vi "get time stamp.vi"(8 "error in (no error)":errorcluster, 10 "clockspeed":dbl, 11 "Image":T1) -> (0 "error out":errorcluster, 3 "timestamp":dbl)   [LabVIEW 2020, in "Point Grey Camera.lvclass"]
uses:
  Point Grey Camera.lvclass
  IMAQ Image.ctl
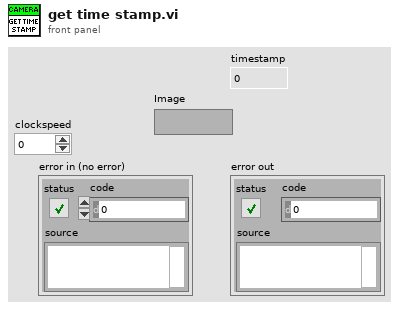
[diagram p1: front panel]
types:
  T1 = typedef "IMAQ Image.ctl" = refnum<image>
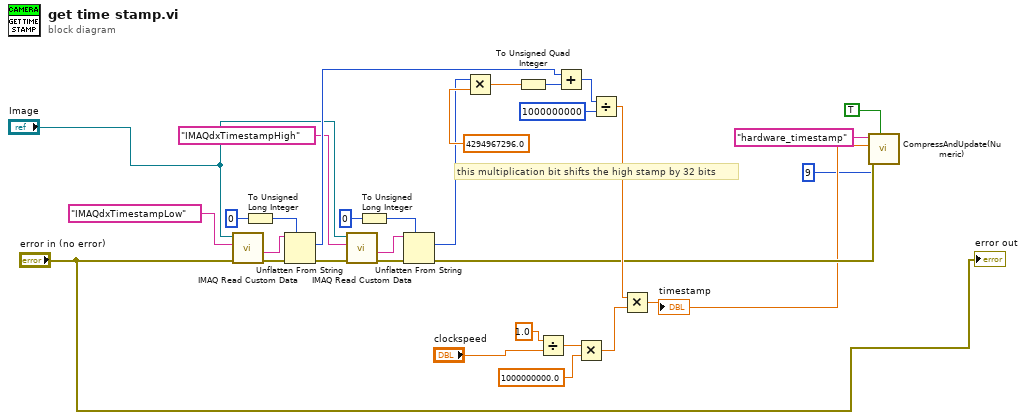
[diagram p0: block diagram]
diagram:
  # "this multiplication bit shifts the high stamp by 32 bits"
  n1 = call "IMAQ Read Custom Data"("error in (no error)"="error in (no error)", "Key"="IMAQdxTimestampLow", "Image"="Image") -> ("error out"=w30:errorcluster, "Custom Data Out"=w17:string)  [unwired: 6 in, 1 out]
  n2 = To Unsigned Long Integer(number=u32 0) -> (unsigned 32bit integer=w16:u32)
  n3 = Unflatten From String(type=w16, binary string=w17, error in (no error)=w30) -> (value=w24:u32, error out=w31:errorcluster)  [unwired: 2 in, 1 out]
  n4 = call "IMAQ Read Custom Data"("error in (no error)"=w31, "Key"="IMAQdxTimestampHigh", "Image"="Image") -> ("error out"=w29:errorcluster, "Custom Data Out"=w20:string)  [unwired: 6 in, 1 out]
  n5 = To Unsigned Long Integer(number=u32 0) -> (unsigned 32bit integer=w19:u32)
  n6 = Unflatten From String(type=w19, binary string=w20, error in (no error)=w29) -> (value=w21:u32, error out=w8:errorcluster)  [unwired: 2 in, 1 out]
  n7 = Multiply(x=w21, y=4294967296.0) -> (x*y=w23:dbl)
  n8 = To Unsigned Quad Integer(1:w23) -> (0:w25:u64)
  n9 = Divide(x=1.0, y="clockspeed") -> (x/y=w11:dbl)
  n10 = Add(x=w24, y=w25) -> (x+y=w26:u64)
  n11 = Multiply(x=w11, y=1000000000.0) -> (x*y=w9:dbl)
  n12 = Divide(x=w26, y=u64 1000000000) -> (x/y=w28:dbl)
  n13 = Multiply(x=w28, y=w9) -> (x*y=w6:dbl)
  "timestamp" <- w6
  n14 = call "CompressAndUpdate(Numeric).vi"("force CVT update (false)"=TRUE, "error in"=w8, "precision (6)"=i16 9, "Numeric"=w6, "command or variable name"="hardware_timestamp") -> ()  [unwired: 6 in, 1 out]
  "error out" <- "error in (no error)"
